vi "绘制方块.vi"(8 "绘制/清除":bool, 9 "网格大小":dbl, 10 "输入点":cluster{"x":dbl, "y":dbl}, 11 "picture":picture caption="图片") -> (3 "new picture":picture caption="新图片")   [LabVIEW 2012]
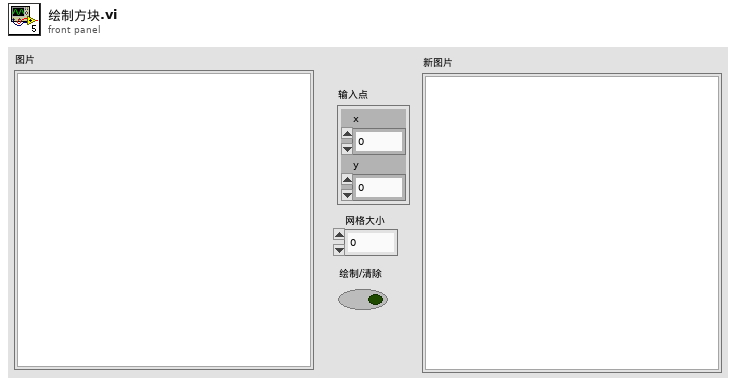
[diagram p1: front panel]
types:
  T1 = cluster{"Width":i16, "Style":enum32{"Solid", "Dash", "Dot", "DashDot", "DashDotDot"}}
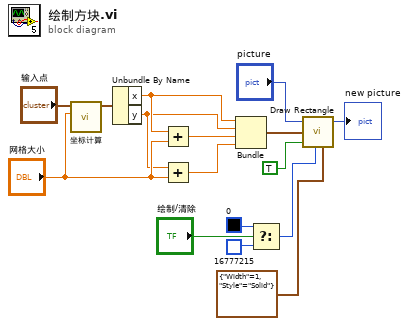
[diagram p0: block diagram]
diagram:
  n1 = call "坐标计算.vi"("网格大小"="网格大小", "输入"="输入点") -> ("输出"=w7:cluster{"x":dbl, "y":dbl})  [unwired: 9 in]
  n2 = Unbundle By Name(w7) -> ("x"=w5:dbl, "y"=w4:dbl)
  n3 = Add(x=w5, y="网格大小") -> (x+y=w3:dbl)
  n4 = Add(x=w4, y="网格大小") -> (x+y=w2:dbl)
  n5 = Bundle("x"=w5, "y"=w4, w3, w2) -> (w1:cluster{"x":dbl, "y":dbl, dbl, dbl})  [unwired: 1 in]
  n6 = Select(t=u32 0 ("color(black)"), s="绘制/清除", f=u32 16777215 ("color(black)")) -> (s? t:f=w9:u32)
  n7 = call <vilib>:"Draw Rectangle.vi"("picture"="picture", "rect"=w1, "fill?(F)"=TRUE, "color(black)"=w9, "pen"=T1 {"Width"=1, "Style"=enum."Solid"}) -> ("new picture"=→"new picture":picture)  [unwired: 4 in]
